vi "smooth IV data.vi"(10 "smooth n":i32, 11 "Array in":dbl[][](array[numeric])) -> (3 "Array out":dbl[][](array[numeric]))   [LabVIEW 2024]
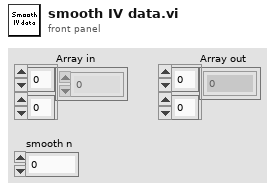
[diagram p1: front panel]
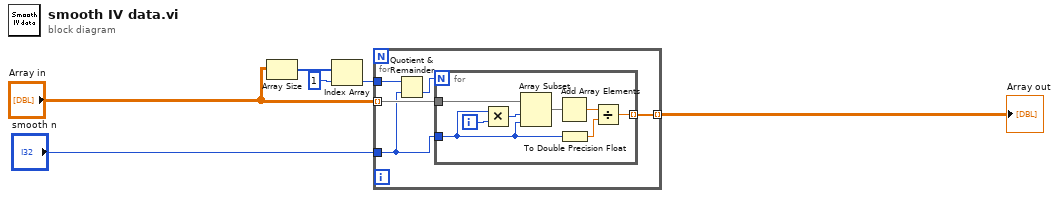
[diagram p0: block diagram]
diagram:
  n1 = Array Size(array="Array in") -> (size(s)=w4:i32[])
  n2 = Index Array(array=w4, index=1) -> (element=w5:i32)
  n3 = for {
    tunnel: "Array in" -> [w9] mode=indexing
    tunnel: "smooth n" -> [w8]
    tunnel: w5 -> [w11]
    tunnel: [w7] -> w2 mode=indexing
    n4 = Quotient & Remainder(x=w11, y=w8) -> (floor(x/y)=w10:i32)  [unwired: 1 out]
    n5 = for {
      N: w10 -> [_]
      tunnel: w9 -> [w19]
      tunnel: w8 -> [w14]
      tunnel: [w12] -> w7 mode=indexing
      i -> [w18]
      n6 = Multiply(x=w14, y=w18) -> (x*y=w17:i32)
      n7 = Array Subset(array=w19, index=w17, length=w14) -> (w16:dbl[])
      n8 = Add Array Elements(numeric array=w16) -> (sum=w15:dbl)
      n9 = To Double Precision Float(number=w14) -> (double precision float=w13:dbl)
      n10 = Divide(x=w15, y=w13) -> (x/y=w12:dbl)
    }
  }
  "Array out" <- w2
